vi "Sine wavegraph.vi"() -> ()   [LabVIEW 2015]
panel:
  out "Waveform Graph":waveform(dbl)(graph)
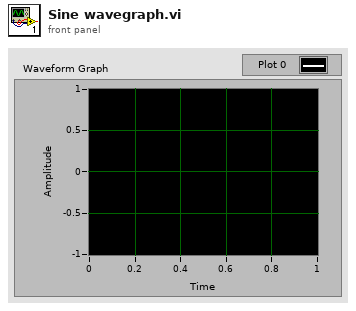
[diagram p1: front panel]
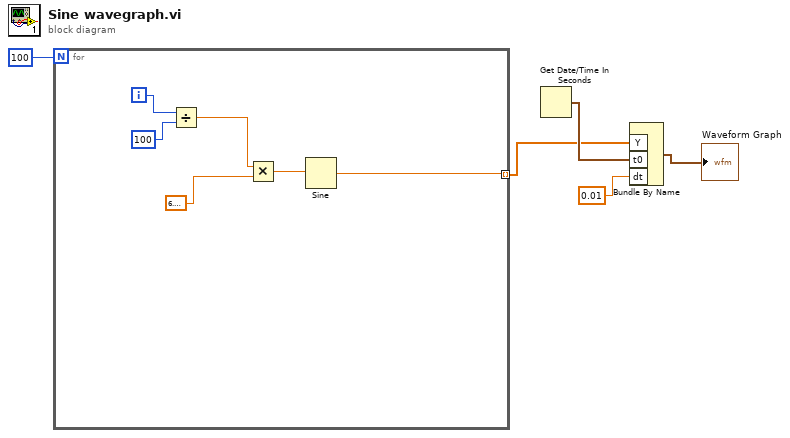
[diagram p0: block diagram]
diagram:
  n1 = for {
    N: 100 -> [_]
    tunnel: [w6] -> w2 mode=indexing
    i -> [w10]
    n2 = Divide(x=w10, y=100) -> (x/y=w8:dbl)
    n3 = Multiply(x=w8, y=6.283185307179586) -> (x*y=w7:dbl)
    n4 = Sine(x=w7) -> (sin(x)=w6:dbl)
  }
  n5 = Get Date/Time In Seconds() -> (seconds since 1Jan1904=w4:timestamp)
  n6 = Bundle By Name("Y"=w2, "t0"=w4, "dt"=0.01) -> (→"Waveform Graph":waveform(dbl))  [unwired: 1 in]
